vi "Get Packed Info.vi"(11 "Data Encoding In":T1) -> (3 "Packed Data Encoding":T1)   [LabVIEW 2021, in "CIF_NI_CIPC.lvlib"]
doc: "Packed data can be transmitted or logged with reduced size. This will create a new data encoding for packed data."
uses:
  CIF_NI_CIPC.lvlib
  TypeDefs/Data Encoding.ctl
  TypeDefs/Alignment.ctl
  <vilib>/CIF Foundation/CIF Utilities/DataTypes/Typedef/Endian.ctl
  TypeDefs/Data Struct Array Info.ctl
  TypeDefs/Data Element.ctl
  <vilib>/Utility/Data Type/Type Definitions/Data Type.ctl
  <vilib>/CIF Foundation/CIF Utilities/DataTypes/DataTypes_CIF_U.lvlib
  <vilib>/Utility/Data Type/NI_Data Type.lvlib
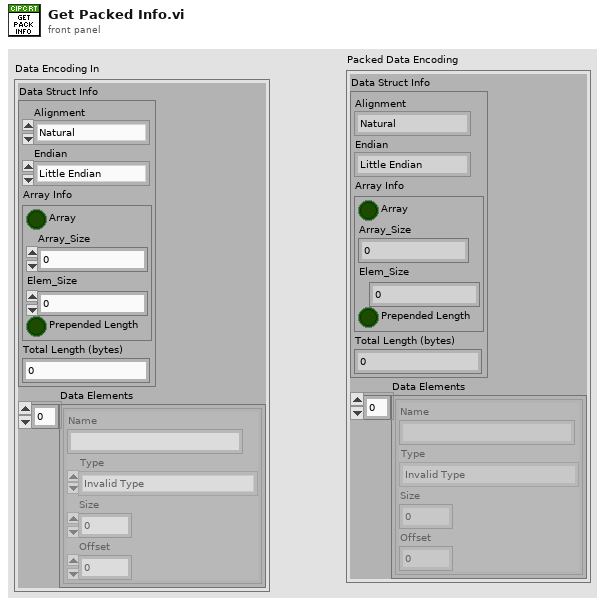
[diagram p1: front panel]
types:
  T1 = typedef "CIF_NI_CIPC.lvlib/Data Encoding.ctl" = cluster{"Data Struct Info":cluster{"Alignment":T2, "Endian":T3, "Array Info":T4, "Total Length (bytes)":i32}, "Data Elements":T5[]}
  T2 = typedef "CIF_NI_CIPC.lvlib/Alignment.ctl" = enum16{"Natural", "Packed"}
  T3 = typedef "DataTypes_CIF_U.lvlib/Endian.ctl" = enum16{"Little Endian", "Big Endian"}
  T4 = typedef "CIF_NI_CIPC.lvlib/Data Struct Array Info.ctl" = cluster{"Array":bool, "Array_Size":i32, "Elem_Size":i32, "Prepended Length":bool}
  T5 = typedef "CIF_NI_CIPC.lvlib/Data Element.ctl" = cluster{"Name":string, "Type":T6, "Size":u32, "Offset":u32}
  T6 = typedef "NI_Data Type.lvlib/Data Type.ctl" = enum8{"Invalid Type", "Void", "I8", "I16", "I32", "I64", "U8", "U16", "U32", "U64", "Single Float", "Double Float", "Extended Float", "Single Complex", "Double Complex", "Extended Complex", "Enum U8", "Enum U16", "Enum U32", "Enum U64", "Single Float With Unit", "Double Float With Unit", "Extended Float With Unit", "Single Complex with Unit", "Double Complex with Unit", "Extended Complex with Unit", "Boolean", "String", "Path", "Picture", "Tag", "Array", "Cluster", "Variant", "LV Variant", "Waveform", "Timestamp", "Digital Waveform", "Digital Data", "ExpressData", "Refnum", "External Data", "VI", "Poly VI", "LabVIEW Class Instance", "Fixed Point", "Set Collection", "Map Collection"}
  T7 = cluster{"Alignment":T2, "Endian":T3, "Array Info":T4, "Total Length (bytes)":i32}
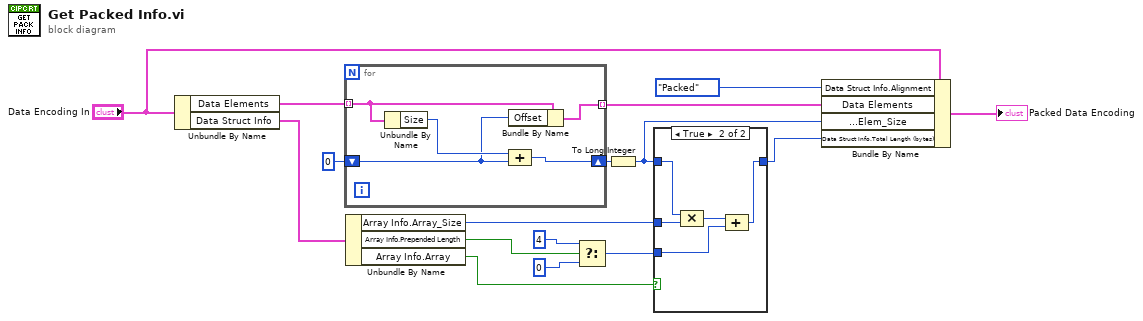
[diagram p0: block diagram]
diagram:
  n1 = Unbundle By Name("Data Encoding In") -> ("Data Elements"=w16:T5[], "Data Struct Info"=w4:T7)
  n2 = for {
    tunnel: w16 -> [w21] mode=indexing
    shift-right: [w20] -> w9
    shift-left: u32 0 ("32bit integer") -> [w17]
    tunnel: [w18] -> w1 mode=indexing
    n3 = Unbundle By Name(w21) -> ("Size"=w19:u32)
    n4 = Bundle By Name(cluster=w21, "Offset"=w17) -> (w18:T5)
    n5 = Compound Arithmetic op=ADD(w19, w17) -> (w20:u32)
  }
  n6 = Unbundle By Name(w4) -> ("Array Info.Array_Size"=w8:i32, "Array Info.Prepended Length"=w15:bool, "Array Info.Array"=w2:bool)
  n7 = Select(t=4 ("32bit integer"), s=w15, f=0 ("32bit integer")) -> (s? t:f=w7:i32)
  n8 = To Long Integer(number=w9) -> (32bit integer=w6:i32)
  n9 = case shown="True" w2 {
    tunnel: w8 -> [_ w27]
    tunnel: w7 -> [_ w25]
    tunnel: w6 -> [w22 w24]
    tunnel: [w22 w23] -> w5
    frame False {
    }
    frame True {
      n10 = Compound Arithmetic op=MULTIPLY(w24, w27) -> (w26:i32)
      n11 = Compound Arithmetic op=ADD(w26, w25) -> (w23:i32)
    }
  }
  n12 = Bundle By Name(cluster="Data Encoding In", "Data Struct Info.Alignment"=Alignment."Packed" ("Array Data Element.Alignment"), "Data Elements"=w1, "Data Struct Info.Array Info.Elem_Size"=w6, "Data Struct Info.Total Length (bytes)"=w5) -> (→"Packed Data Encoding":T1)
